vi "Front Panel Magic.vi"(6 "Variant in":variant, 7 "Shift Pressed?":bool, 8 "error in (no error)":errorcluster, 10 "QD Combo Box Ref":refnum<vi>, 11 "QD Launch VI Ref":refnum<vi>) -> (0 "error out":errorcluster, 4 "Variant out":variant)   [LabVIEW 2017]
doc: "This quick drop plugin is designed to clean up the front panel of non UI VIs.\n\nThis magic includes:\nAuto naming of class inputs and outputs that are wired to the front panel.\nStandardizing of the error cluster inputs and outputs if they exist.\nAlligning all front panel items to their corresponding spots on the connector pane.\n\nThis plugin is not intended for use on user interface VIs and will have no effect if it is called on a VI with UI somewhere in its title.\n\nDefault Shortcut - [$A]"
uses:
  <vilib>/regexp/Match Regular Expression.xnode
panel:
  # "Do not change the connector pane of this VI.\n\nSee the block diagram for directions on how to use this template."
  # "Specify the name of the Undo transaction"
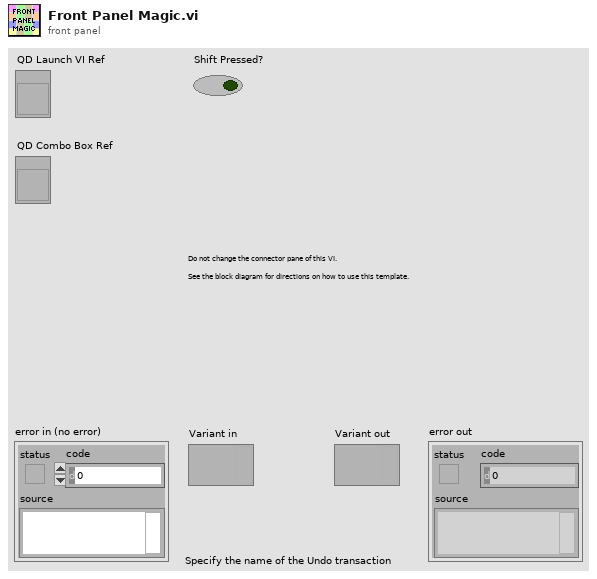
[diagram p1: front panel]
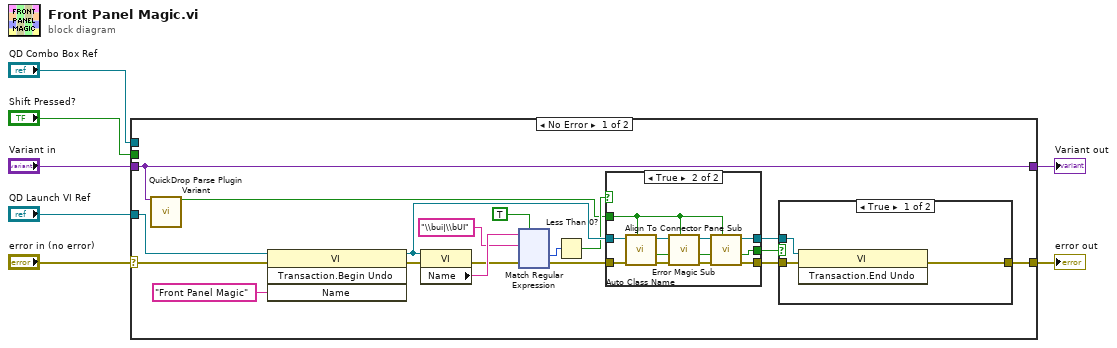
[diagram p0: block diagram]
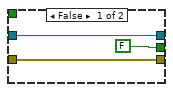
[diagram p2: hidden frame]
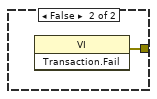
[diagram p3: hidden frame]
diagram:
  n1 = case shown="No Error" "error in (no error)" {
    selector: "error in (no error)" -> [w25 w160]
    tunnel: [w22 w160] -> w6
    tunnel: "QD Launch VI Ref" -> [w23 _]
    tunnel: "Shift Pressed?" -> [_ _]
    tunnel: "QD Combo Box Ref" -> [_ _]
    tunnel: "Variant in" -> [w24 w159]
    tunnel: [w24 w159] -> w1
    frame No Error {
      n2 = call <vilib>:"QuickDrop Parse Plugin Variant.vi"("QDKS Variant in"=w24) -> ("QD Launch VI Panel?"=w8:bool)  [unwired: 12 in, 2 out]
      n3 = invoke class="VI" method="Transaction.Begin Undo"(reference=w23, error in=w25, "Name"="Front Panel Magic") -> (reference out=w13:refnum<vi>, error out=w12:errorcluster)  [unwired: 1 in, 2 out]
      n4 = property class="VI"(reference=w13, error in=w12) -> (error out=w14:errorcluster, "Name"=w17:string)  [unwired: 1 out]
      n5 = xnode "Match Regular Expression"("input string"=w17, "regular expression"="\\bui|\\bUI", "error in"=w14, "ignore case? (F)"=TRUE) -> ("offset past match"=w11:i32, "error out"=w9:errorcluster)  [unwired: 2 in, 3 out]
      n6 = Less Than 0?(x=w11) -> (x < 0?=w10:bool)
      n7 = case shown="True" w10 {
        tunnel: [w28 w40] -> w20
        tunnel: [w27 w39] -> w19
        tunnel: [FALSE w30] -> w18
        tunnel: w13 -> [w27 w38]
        tunnel: w9 -> [w28 w37]
        tunnel: w8 -> [_ w29]
        frame False {
        }
        frame True {
          n8 = call "Auto Class Name.vi"("QD Launch VI Panel?"=w29, "error in (no error)"=w37, "VI in"=w38) -> ("error out"=w33:errorcluster, "Changed Out"=w32:bool, "VI out"=w36:refnum<vi>)  [unwired: 6 in]
          n9 = call "Error Magic Sub.vi"("QD Launch VI Panel?"=w29, "error in (no error)"=w33, "Changed In"=w32, "VI in"=w36) -> ("error out"=w34:errorcluster, "Changed Out"=w31:bool, "VI out"=w35:refnum<vi>)  [unwired: 5 in]
          n10 = call "Align To Connector Pane Sub.vi"("QD Launch VI Panel?"=w29, "error in (no error)"=w34, "Changed In"=w31, "VI in"=w35) -> ("error out"=w40:errorcluster, "Changed Out"=w30:bool, "VI out"=w39:refnum<vi>)  [unwired: 5 in]
        }
      }
      n11 = case shown="True" w18 {
        tunnel: [w157 w158] -> w22
        tunnel: w20 -> [w156 _]
        tunnel: w19 -> [w155 _]
        frame True {
          n12 = invoke class="VI" method="Transaction.End Undo"(reference=w155, error in=w156) -> (error out=w157:errorcluster)  [unwired: 1 in, 2 out]
        }
        frame False {
          n13 = invoke class="VI" method="Transaction.Fail"() -> (error out=w158:errorcluster)  [unwired: 3 in, 2 out]
        }
      }
    }
    frame Error {
    }
  }
  "error out" <- w6
  "Variant out" <- w1
